vi "get Config.vi"(11 "Ship in":refnum<class "Ship.lvclass">) -> (3 "Common":T1)   [LabVIEW 2021, in "Ship.lvclass"]
uses:
  Ship.lvclass
  Ship.lvclass/Ship.ctl
  Config.ctl
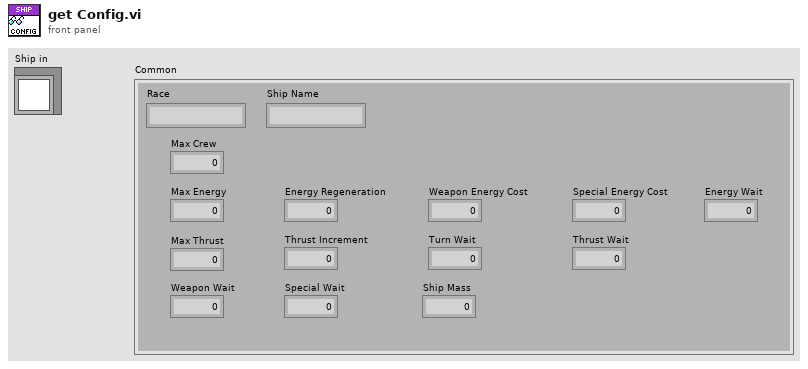
[diagram p1: front panel]
types:
  T1 = typedef "Ship.lvclass/Config.ctl" = cluster{"Race":string, "Ship Name":string, "Max Crew":i32, "Max Energy":i32, "Energy Regeneration":i32, "Weapon Energy Cost":i32, "Special Energy Cost":i32, "Energy Wait":i32, "Max Thrust":i32, "Thrust Increment":i32, "Turn Wait":i32, "Thrust Wait":i32, "Weapon Wait":i32, "Special Wait":i32, "Ship Mass":i32}
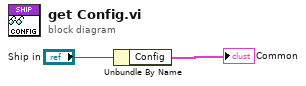
[diagram p0: block diagram]
diagram:
  n1 = Unbundle By Name("Ship in") -> ("Config"=→"Common":T1)
